vi "Write Status 1D.vi"(8 "error in (no error)":errorcluster, 10 "status":T1[](array[typedef]), 11 "Transfer Group Status in":refnum<class "Transfer Group Status.lvclass">) -> (0 "error out":errorcluster, 3 "Transfer Group Status out":refnum<class "Transfer Group Status.lvclass">)   [LabVIEW 2017, in "DSF Core.lvlib" / "Transfer Group Status.lvclass"]
uses:
  Transfer Group Status.lvclass
  C:/Program Files (x86)/National Instruments/LabVIEW 2017/vi.lib/NI/Memory Manager/Classes/Pointer/Pointer.lvclass
  Typedefs/DSF Transfer Group Status.ctl
  <vilib>/NI/Memory Manager/Classes/Pointer/Pointer.lvclass/Pointer.ctl
  <vilib>/NI/Memory Manager/Classes/Pointer/Errors.vi
  <vilib>/NI/Memory Manager/Classes/Pointer/Out of Bounds.vi
  <vilib>/NI/Memory Manager/Classes/Pointer/Get Size.vi
  <vilib>/NI/Memory Manager/VIs/Source.Write.String.vi
  <vilib>/NI/Memory Manager/Classes/Pointer/Write Pointer Size.vi
  <vilib>/NI/Memory Manager/Classes/Pointer/Create Error.vi
  <vilib>/NI/Memory Manager/VIs/Source.Write.Scalar.Base10.vi
  <vilib>/NI/Memory Manager/VIs/Source.Write.Scalar.Base10 (U64).vi
  <vilib>/NI/Memory Manager/VIs/New Error Cluster Constant.vi
  <vilib>/NI/Memory Manager/VIs/New Error Cluster Constant (512B).vi
  <vilib>/NI/Memory Manager/VIs/Error Cluster.Set Status.vi
  <vilib>/NI/Memory Manager/VIs/Error Cluster.Set Code.vi
  <vilib>/NI/Memory Manager/VIs/Error Cluster.Set VI Source.vi
  <vilib>/NI/Memory Manager/Constants/Constants.vi
  <vilib>/NI/Memory Manager/Constants/Library Name.vi
  <vilib>/NI/Memory Manager/Classes/Pointer/Pointer Error Info.vi
  <vilib>/NI/Memory Manager/Constants/Pointer Class Name.vi
  <vilib>/NI/Memory Manager/Classes/Pointer/Pointer.lvclass
  DSF Core.lvlib
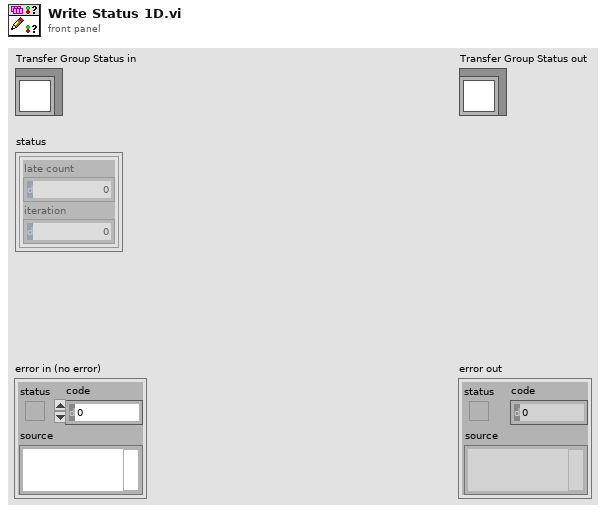
[diagram p1: front panel]
types:
  T1 = typedef "DSF Core.lvlib/DSF Transfer Group Status.ctl" = cluster{"late count":u64, "iteration":u64}
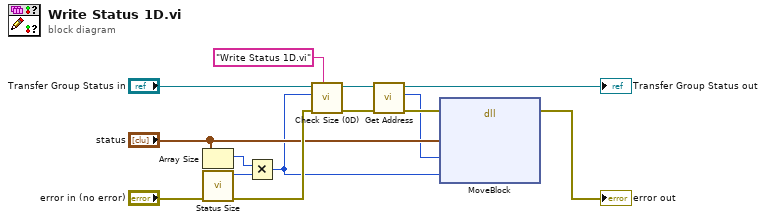
[diagram p0: block diagram]
diagram:
  n1 = Array Size(array="status") -> (size(s)=w4:i32)
  n2 = call "Status Size.vi"("error in (no error)"="error in (no error)") -> ("error out"=w10:errorcluster, "size"=w3:u64)  [unwired: 9 in]
  n3 = Multiply(x=w4, y=w3) -> (x*y=w2:u64)
  n4 = call <vilib>:"Check Size (0D).vi"("source vi name"="Write Status 1D.vi", "error in (no error)"=w10, "required size"=w2, "Pointer in"="Transfer Group Status in") -> ("error out"=w11:errorcluster, "Pointer out"=w13:refnum<class "Transfer Group Status.lvclass">)  [unwired: 5 in, 1 out]
  n5 = call <vilib>:"Get Address.vi"("Pointer in"=w13) -> ("address"=w1:u64, "Pointer out"=→"Transfer Group Status out":refnum<class "Transfer Group Status.lvclass">)  [unwired: 9 in]
  n6 = dll-call lib="LabVIEW" fn="MoveBlock"(error in=w11, "src"="status", "dst"=w1, "size"=w2) -> (error out=→"error out":errorcluster)  [unwired: 6 in, 1 out]
